vi "Get Name.vi"(11 "Plugin in":refnum<class "Plugin.lvclass">) -> (2 "name":string, 3 "Plugin out":refnum<class "Plugin.lvclass">)   [LabVIEW 2017, in "DSF Core.lvlib" / "Plugin.lvclass"]
uses:
  Plugin.lvclass
  Plugin.lvclass/Plugin.ctl
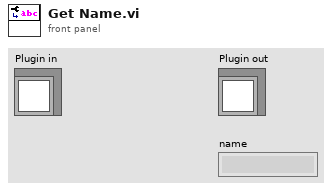
[diagram p1: front panel]
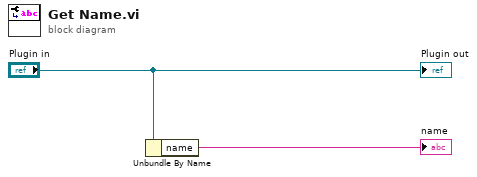
[diagram p0: block diagram]
diagram:
  n1 = Unbundle By Name("Plugin in") -> ("name"=→"name":string)
  "Plugin out" <- "Plugin in"
